vi "ToteCount.vi"() -> ()   [LabVIEW 2014]
panel:
  in  "ToteCount":i32
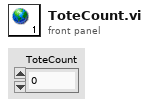
[diagram p1: front panel]
diagram:
